vi "destroy user events.vi"(8 "error in (no error)":errorcluster, 11 "DataGridView in":refnum<class "DataGridView.lvclass">) -> (0 "error out":errorcluster)   [LabVIEW 2013, in "DataGrid.lvlib" / "DataGridView.lvclass"]
uses:
  DataGridView.lvclass
  DataGridView.lvclass/DataGridView.ctl
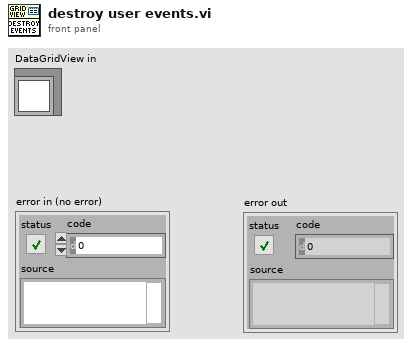
[diagram p1: front panel]
types:
  T1 = cluster{"CellClicked":refnum<user-event>, "CellValue Changed":refnum<user-event>, "KeyDown":refnum<user-event>, "DataError":refnum<user-event>, "UserAddedRow":refnum<user-event>, "UserDeletedRow":refnum<user-event>}
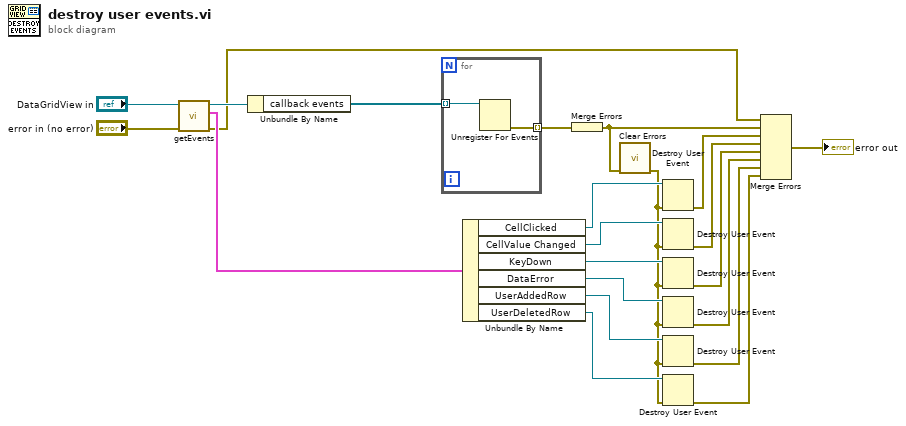
[diagram p0: block diagram]
diagram:
  n1 = call "getEvents.vi"("error in (no error)"="error in (no error)", "DataGridView in"="DataGridView in") -> ("error out"=w8:errorcluster, "userEvents"=w17:T1, "DataGridView out"=w18:refnum<class "DataGridView.lvclass">)  [unwired: 7 in]
  n2 = Unbundle By Name(w18) -> ("callback events"=w22:refnum<k27>[])
  n3 = for {
    tunnel: w22 -> [w24] mode=indexing
    tunnel: [w23] -> w21 mode=indexing
    n4 = Unregister For Events(event registration refnum=w24) -> (error out=w23:errorcluster)  [unwired: 1 in]
  }
  n5 = Unbundle By Name(w17) -> ("CellClicked"=w16:refnum<user-event>, "CellValue Changed"=w15:refnum<user-event>, "KeyDown"=w14:refnum<user-event>, "DataError"=w13:refnum<user-event>, "UserAddedRow"=w12:refnum<user-event>, "UserDeletedRow"=w11:refnum<user-event>)
  n6 = Merge Errors(w21) -> (w7:errorcluster)
  n7 = call <vilib>:"Clear Errors.vi"("error in (no error)"=w7) -> ("error out"=w10:errorcluster)  [unwired: 6 in]
  n8 = Destroy User Event(user event=w16, error in=w10) -> (error out=w6:errorcluster)
  n9 = Destroy User Event(user event=w15, error in=w10) -> (error out=w5:errorcluster)
  n10 = Destroy User Event(user event=w14, error in=w10) -> (error out=w4:errorcluster)
  n11 = Destroy User Event(user event=w13, error in=w10) -> (error out=w3:errorcluster)
  n12 = Destroy User Event(user event=w12, error in=w10) -> (error out=w2:errorcluster)
  n13 = Destroy User Event(user event=w11, error in=w10) -> (error out=w1:errorcluster)
  n14 = Merge Errors(w8, w7, w6, w5, w4, w3, w2, w1) -> (→"error out":errorcluster)
